vi "GEOM_ReadType.vi"(6 "override format":string, 8 "error in (no error)":errorcluster, 10 "TYPE":string, 11 "database path":path=path "/home/ArcVIEW/Modules/Geometry/database") -> (0 "error out":errorcluster, 1 "format out":string, 2 "Detector":cluster{"Info":string[][], "ReadModes":T1[]} {"ReadModes"."amplifiers"."fliped" items=["none", "horizontal", "vertical"]; "ReadModes"."amplifiers"."type" items=["LL", "LR", "UL", "UR"]}, 3 "database path out":path=path "/home/ArcVIEW/Modules/Geometry/database/TYPES/Hawaii-II_4ch.chp")   [LabVIEW 2016]
uses:
  GEOM_ReadMode.ctl
  GEOM_Amplifier.ctl
  GEOM_AmpType.ctl
  GEOM_ROI.ctl
  GEOM_Coords.ctl
panel:
  in  "ReadMode":T1 {"amplifiers"."fliped" items=["none", "horizontal", "vertical"]; "amplifiers"."type" items=["LL", "LR", "UL", "UR"]}
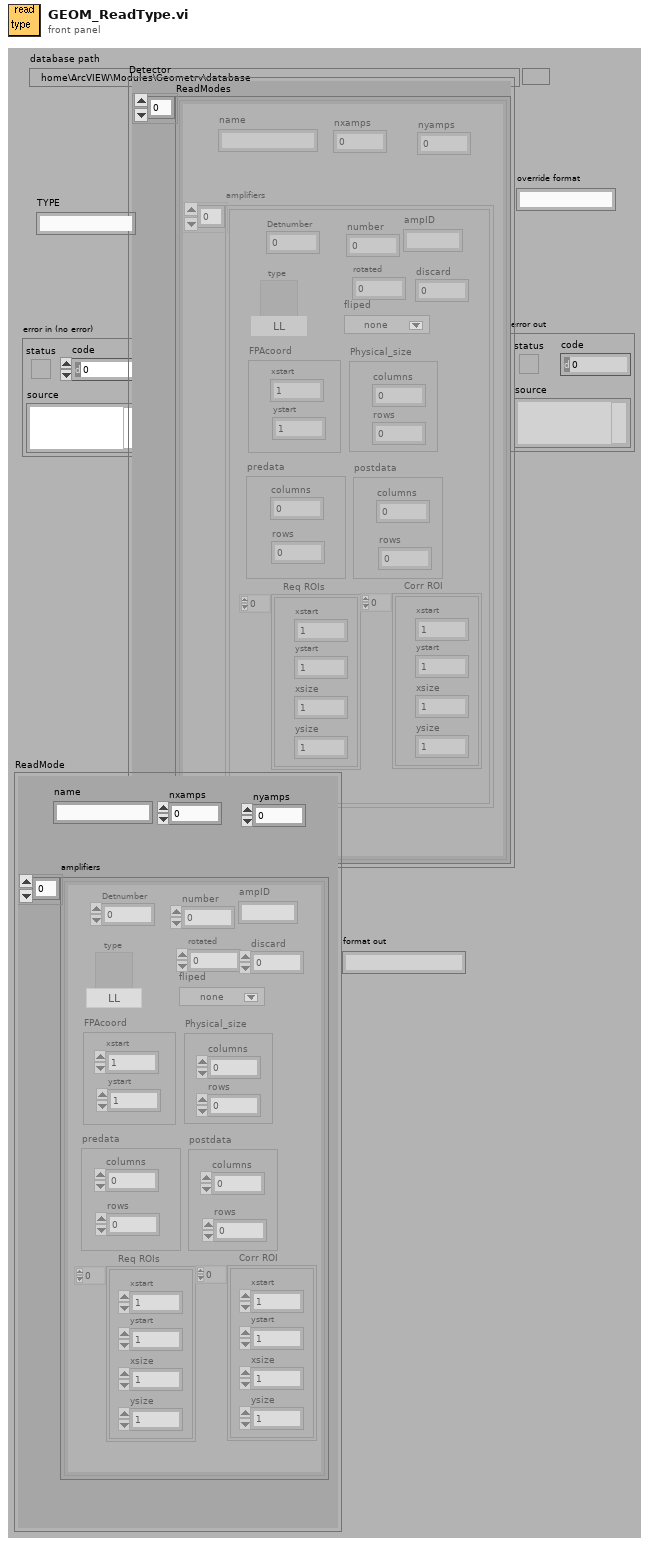
[diagram p1: front panel]
types:
  T1 = typedef "GEOM_ReadMode.ctl" = cluster{"name":string, "amplifiers":T2[], "nxamps":i32, "nyamps":i32}
  T2 = typedef "GEOM_Amplifier.ctl" = cluster{"number":i32, "type":T3, "rotated":i16, "fliped":u16, "FPAcoord":cluster{"xstart":i32, "ystart":i32}, "Physical_size":cluster{"columns":i32, "rows":i32}, "predata":cluster{"columns":i32, "rows":i32}, "postdata":cluster{"columns":i32, "rows":i32}, "Req ROIs":T4, "Corr ROI":T4, "Detnumber":i32, "ampID":string, "discard":i32}
  T3 = typedef "GEOM_AmpType.ctl" = u16
  T4 = typedef "GEOM_ROI.ctl" = T5[]
  T5 = typedef "GEOM_Coords.ctl" = cluster{"xstart":u32, "ystart":u32, "xsize":u32, "ysize":u32}
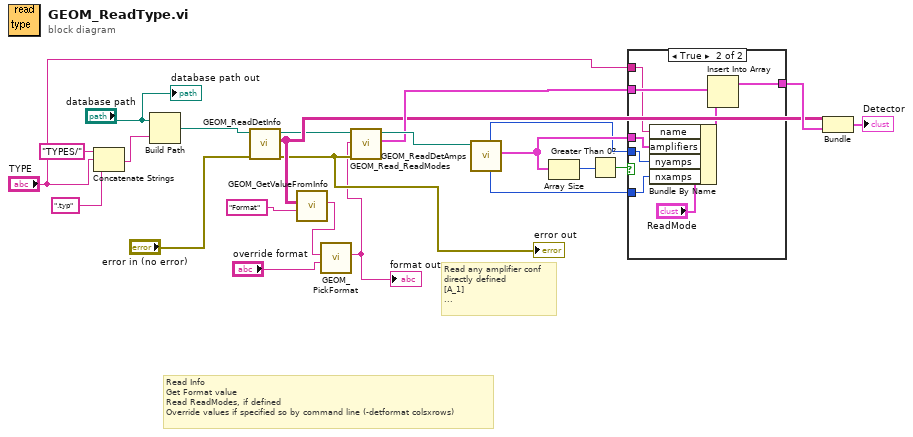
[diagram p0: block diagram]
diagram:
  # "Read any amplifier conf\ndirectly defined\n[A_1]\n..."
  # "Read Info\nGet Format value\nRead ReadModes, if defined\nOverride values if specified so by command line (-detformat colsxrows)"
  n1 = Concatenate Strings("TYPES/" ("string"), "TYPE", ".typ" ("regular expression")) -> (w10:string)
  n2 = Build Path(base path="database path", name or relative path=w10) -> (appended path=w9:path)
  n3 = call "GEOM_ReadDetInfo.vi"("error in (no error)"="error in (no error)", "file path"=w9) -> ("error out"=w13:errorcluster, "Info"=w15:string[][], "file path out"=w6:path)  [unwired: 7 out]
  "error out" <- w13
  n4 = call "GEOM_GetValueFromInfo.vi"("Key"="Format", "Info"=w15) -> ("Value"=w2:string)  [unwired: 9 out]
  n5 = call "GEOM_PickFormat.vi"("requested format"="override format", "default format in"=w2) -> ("format out"=w1:string)  [unwired: 9 out]
  "format out" <- w1
  n6 = call "GEOM_Read_ReadModes.vi"("error in (no error)"=w13, "Detector Format"=w1, "file path"=w6) -> ("ReadModes"=w21:T1[], "file path out"=w22:path)  [unwired: 7 out]
  n7 = call "GEOM_ReadDetAmps.vi"("file path"=w22) -> ("amplifiers"=w18:T2[], "numxamps"=w5:i32, "numyamps"=w4:i32)  [unwired: 3 in, 5 out]
  n8 = Array Size(array=w18) -> (size(s)=w17:i32)
  n9 = Greater Than 0?(x=w17) -> (x > 0?=w16:bool)
  n10 = case shown="True" w16 {
    tunnel: w21 -> [w24 w32]
    tunnel: "TYPE" -> [_ w28]
    tunnel: w18 -> [_ w27]
    tunnel: [w24 w30] -> w20
    tunnel: w5 -> [_ w26]
    tunnel: w4 -> [_ w25]
    frame False {
    }
    frame True {
      n11 = Bundle By Name(cluster="ReadMode", "name"=w28, "amplifiers"=w27, "nyamps"=w25, "nxamps"=w26) -> (w31:T1)
      n12 = Insert Into Array(array=w32, new element=w31) -> (w30:T1[])  [unwired: 1 in]
    }
  }
  n13 = Bundle("Info"=w15, "ReadModes"=w20) -> (→"Detector":cluster{"Info":string[][], "ReadModes":T1[]})  [unwired: 1 out]
  "database path out" <- "database path"
